vi "Process Channel.vi"(8 "error in":errorcluster, 11 "WaveformProcessor":refnum<class "WaveformProcessor.lvclass">) -> (0 "error out":errorcluster, 3 "WaveformProcessor out":refnum<class "WaveformProcessor.lvclass">)   [LabVIEW 2019, in "Variant Parser.lvlib" / "WaveformProcessor.lvclass"]
uses:
  Library/WaveformProcessor.lvclass
  Library/WaveformProcessor.lvclass/WaveformProcessor.ctl
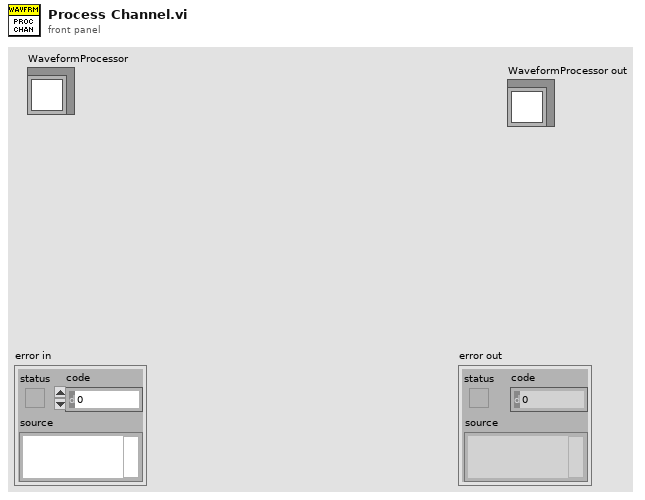
[diagram p1: front panel]
types:
  T1 = typedef "Variant Parser.lvlib/WaveformProcessor.lvclass/Pulse Analysis.ctl" = cluster{"tpulseStart":dbl, "tpulseEnd":dbl, "RisingSlope":dbl, "FallingSlope":dbl, "tHoldoff":dbl, "PeakAmplitude":dbl, "PulseAmplitude":dbl, "tpulse":dbl, "tPulseRise":dbl, "tPulseFall":dbl}
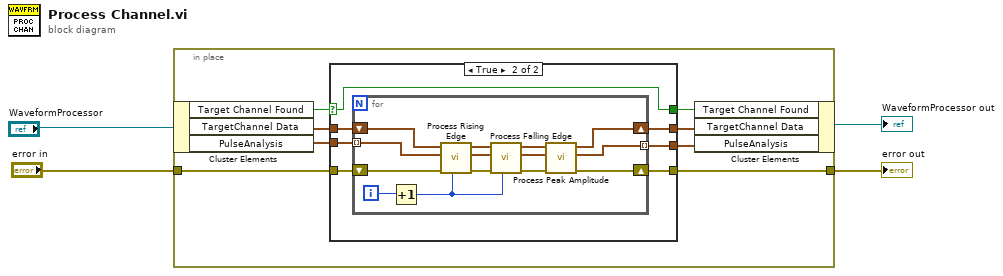
[diagram p0: block diagram]
diagram:
  n1 = in-place {
    in-place-border: "error in" -> [w8]
    in-place-border: [w7] -> w3
    n2 = in-place-cluster #1("WaveformProcessor") -> ("Target Channel Found"=w6:bool, "TargetChannel Data"=w12:waveform(dbl), "PulseAnalysis"=w10:T1[])
    n3 = case shown="True" w6 {
      selector: w6 -> [w16 w17]
      tunnel: w12 -> [w15 w23]
      tunnel: [w15 w22] -> w11
      tunnel: w10 -> [w14 w21]
      tunnel: [w14 w20] -> w9
      tunnel: w8 -> [w13 w19]
      tunnel: [w13 w18] -> w7
      tunnel: [w16 w17] -> w5
      frame False {
      }
      frame True {
        n4 = for {
          shift-right: [w25] -> w22
          shift-left: w23 -> [w37]
          tunnel: w21 -> [w36] mode=indexing
          tunnel: [w24] -> w20 mode=indexing
          shift-right: [w26] -> w18
          shift-left: w19 -> [w34]
          i -> [w35]
          n5 = Increment(x=w35) -> (x+1=w30:i32)
          n6 = call "Process Rising Edge.vi"("edge number (1)"=w30, "error in"=w34, "PulseAnalysis in"=w36, "ChannelData in"=w37) -> ("error out"=w33:errorcluster, "PulseAnalysis out"=w32:T1, "ChannelData Out"=w31:waveform(dbl))  [unwired: 5 in]
          n7 = call "Process Falling Edge.vi"("edge number (1)"=w30, "error in"=w33, "PulseAnalysis in"=w32, "ChannelData in"=w31) -> ("error out"=w27:errorcluster, "PulseAnalysis out"=w28:T1, "ChannelData Out"=w29:waveform(dbl))  [unwired: 5 in]
          n8 = call "Process Peak Amplitude.vi"("error in"=w27, "PulseAnalysis in"=w28, "ChannelData in"=w29) -> ("error out"=w26:errorcluster, "PulseAnalysis out"=w24:T1, "ChannelData Out"=w25:waveform(dbl))  [unwired: 6 in]
        }
      }
    }
    n9 = in-place-cluster #1("Target Channel Found"=w5, "TargetChannel Data"=w11, "PulseAnalysis"=w9) -> (→"WaveformProcessor out":refnum<class "WaveformProcessor.lvclass">)
  }
  "error out" <- w3
